vi "Pre Launch Init.vi"(11 "Signal Generation in":refnum<class "Signal Generation.lvclass">) -> (0 "error out":errorcluster, 3 "Signal Generation out":refnum<class "Signal Generation.lvclass">)   [LabVIEW 2020, in "Signal Generation.lvlib" / "Signal Generation.lvclass"]
doc: "(<B>Filename</B>: Actor Framework.lvlib:Actor.lvclass:Pre Launch Init.vi)\n\nDefines behavior that occurs after the Launch Nested Actor method is invoked but before the actor's Actor Core method begins running.\n\nBy default, this method does nothing. A descendant class may override it to define behavior."
uses:
  Signal Generation.lvclass
  Controls/SignalParamTD.ctl
  Controls/SignalShapeTD.ctl
  Signal Generation.lvclass/Signal Generation.ctl
  <vilib>/ActorFramework/Actor/Actor.lvclass
  Signal Generation.lvlib
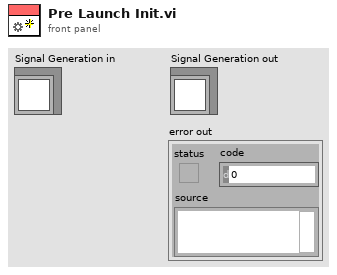
[diagram p1: front panel]
types:
  T1 = typedef "SignalParamTD.ctl" = cluster{"Frequency":u32, "Amplitude":dbl, "Signal Shape":T2}
  T2 = typedef "SignalShapeTD.ctl" = enum16{"Sine", "Square", "Triangle"}
  T3 = cluster{"Start/Stop":refnum<user-event>, "Exit":refnum<user-event>, "Signal Parameters":refnum<user-event>}
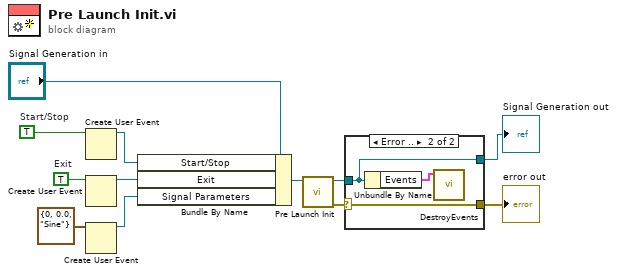
[diagram p0: block diagram]
diagram:
  w11 = TRUE  # Exit
  w12 = TRUE  # Start/Stop
  n1 = Create User Event(user event datatype=w12) -> (user event=w8:refnum<user-event>)  [unwired: 1 in, 1 out]
  n2 = Create User Event(user event datatype=w11) -> (user event=w7:refnum<user-event>)  [unwired: 1 in, 1 out]
  n3 = Create User Event(user event datatype=T1 {"Frequency"=0, "Amplitude"=0.0, "Signal Shape"=enum."Sine"} ("Signal Parameters")) -> (user event=w6:refnum<user-event>)  [unwired: 1 in, 1 out]
  n4 = Bundle By Name(cluster="Signal Generation in", "Start/Stop"=w8, "Exit"=w7, "Signal Parameters"=w6) -> (w9:refnum<class "Signal Generation.lvclass">)
  n5 = call-parent "Pre Launch Init.vi"("Actor in"=w9) -> ("error out"=w4:errorcluster, "Actor out"=w2:refnum<class "Signal Generation.lvclass">)  [unwired: 9 in]
  n6 = case shown="Error .." w4 {
    selector: w4 -> [w14 w15]
    tunnel: [w14 w15] -> w3
    tunnel: w2 -> [w13 w16]
    tunnel: [w13 w16] -> w1
    frame No Error {
    }
    frame Error {
      n7 = Unbundle By Name(w16) -> ("Events"=w17:T3)
      n8 = call "DestroyEvents.vi"("Events"=w17) -> ()  [unwired: 10 in, 1 out]
    }
  }
  "error out" <- w3
  "Signal Generation out" <- w1
